vi "_Close.vi"(8 "error in":errorcluster, 11 "Device In":i32) -> (0 "error out":errorcluster, 3 "Device Out":i32)   [LabVIEW 2014]
uses:
  phidget21.dll
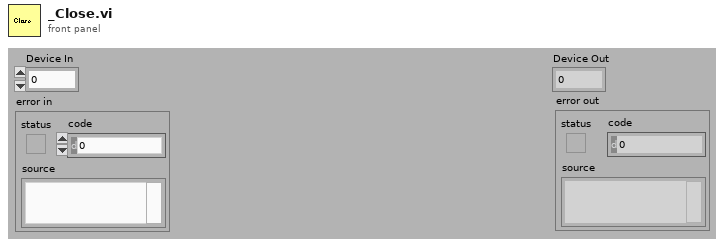
[diagram p1: front panel]
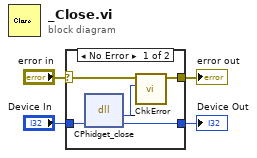
[diagram p0: block diagram]
diagram:
  n1 = case shown="No Error" "error in" {
    selector: "error in" -> [w7 w11]
    tunnel: [w5 w11] -> w3
    tunnel: "Device In" -> [w9 w10]
    tunnel: [w8 w10] -> w1
    frame No Error {
      n2 = dll-call lib="phidget21.*" fn="CPhidget_close"("phid"=w9) -> (w6:i32, "phid"=w8:i32)  [unwired: 3 in, 2 out]
      n3 = call "_ChkError.vi"("Return Code"=w6, "error in (no error)"=w7) -> ("error out"=w5:errorcluster)  [unwired: 9 in]
    }
    frame Error {
    }
  }
  "error out" <- w3
  "Device Out" <- w1
